vi "Search_for_miniScan.vi"(11 "AOL ZStack Path":path) -> (1 "Frame Size":i64, 2 "POI/ROI":bool, 3 "ROI ID":i64)   [LabVIEW 2017]
uses:
  <userlib>/My Palettes.lib/Files & paths/Spreadsheet/Read From Spreadsheet File (I64)-Mod.vi
panel:
  # "True if POI exists"
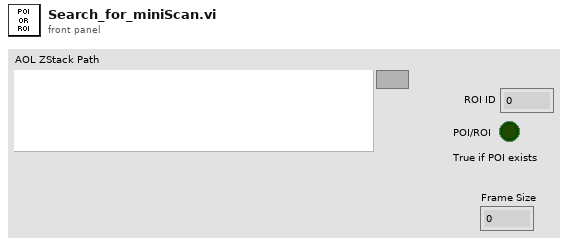
[diagram p1: front panel]
types:
  T1 = typedef "Fixed strings.ctl" = cluster{"ROI file name":string, "Normalised ROI file name":string, "Zplane Pockels values file name":string, "Functional data folder name":string, "Experiment Header file name":string, "Z-stack images folder name":string, "Groups setup rel. path":string, "Groups text file rel. path":string, "TDMS files folder name (F.img)":string, "TDMS files folder name (V.acq)":string, "TDMS files folder name (Pl.acq)":string, "Cycle rel times sequence file":string, "Dynamically called VIs folder name":string, "Time Series folder base name":string}
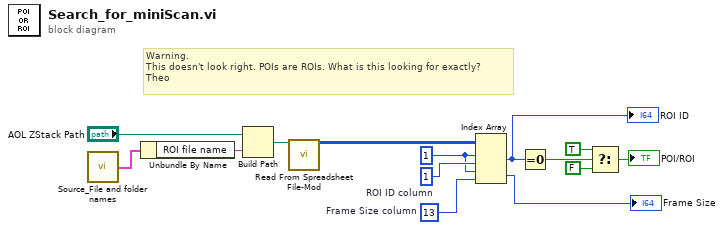
[diagram p0: block diagram]
diagram:
  w2 = 13  # Frame Size column
  w12 = 1  # ROI ID column
  w3 = 1 ("index (row)")
  # "Warning.\nThis doesn't look right. POIs are ROIs. What is this looking for exactly?\nTheo"
  n1 = call "Source_File and folder names.vi"() -> ("Fixed strings"=w5:T1)  [unwired: 1 in]
  n2 = Unbundle By Name(w5) -> ("ROI file name"=w4:string)
  n3 = Build Path(base path="AOL ZStack Path", name or relative path=w4) -> (appended path=w14:path)
  n4 = call-poly <userlib>:"Read From Spreadsheet File-Mod.vi"("file path (dialog if empty)"=w14) -> ("all rows"=w13:i64[][])  [unwired: 9 in, 5 out]
  n5 = Index Array(array=w13, index (row) #1=w3, index (col) #1=w12, index (row) #2=w3, index (col) #2=w2) -> (element #1=w11:i64, element #2=→"Frame Size":i64)
  "ROI ID" <- w11
  n6 = Equal To 0?(x=w11) -> (x = 0?=w10:bool)
  n7 = Select(t=TRUE, s=w10, f=FALSE) -> (s? t:f=→"POI/ROI":bool)
